vi "estimate_frequency.vi"(4 "FFT Length":i32, 5 "State In":sgl[](array[numeric]), 6 "Prediction Lookahead":sgl, 7 "Central Tip Position (KF)":sgl[](array[numeric])) -> (0 "Prediction":dbl, 1 "State Out":sgl[](array[numeric]), 2 "FFT1":cdb[](array[numeric]), 3 "Xarr":sgl[](array[numeric]))   [LabVIEW 2013]
uses:
  <vilib>/Analysis/2dsp.llb/Real FFT.vi
  <vilib>/Analysis/NI_AALPro.lvlib
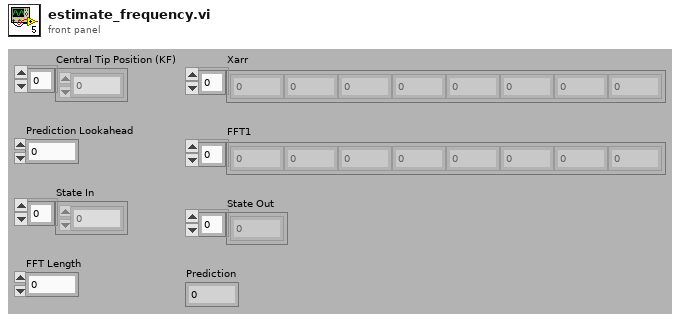
[diagram p1: front panel]
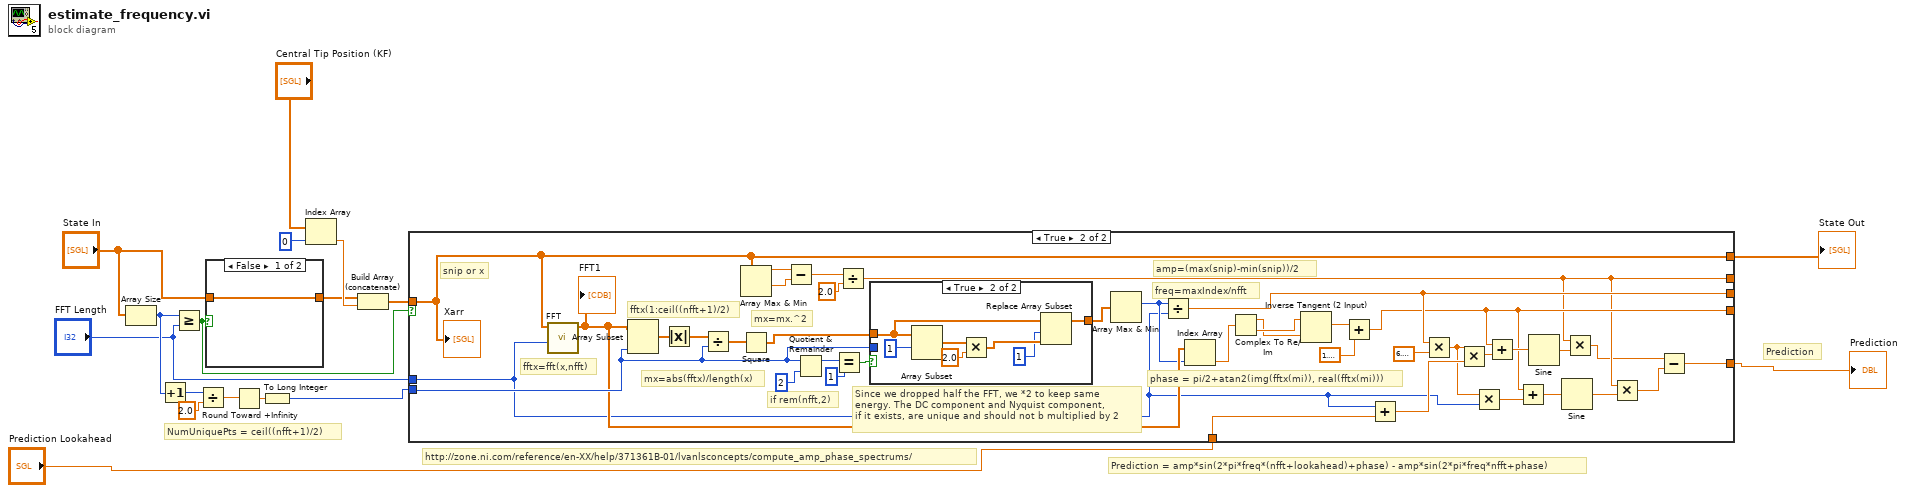
[diagram p0: block diagram]
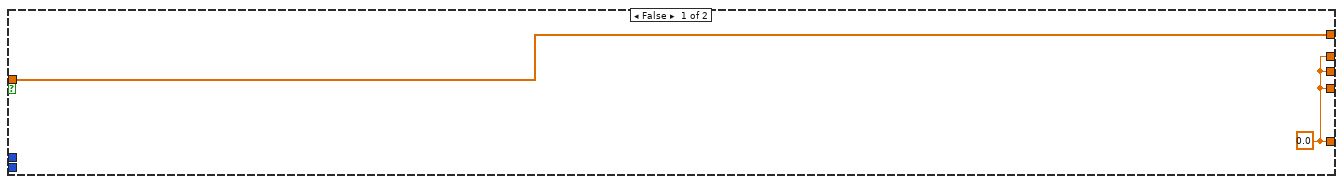
[diagram p2: hidden frame]
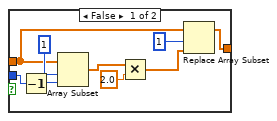
[diagram p3: hidden frame]
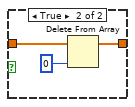
[diagram p4: hidden frame]
diagram:
  # "Prediction = amp*sin(2*pi*freq*(nfft+lookahead)+phase) - amp*sin(2*pi*freq*nfft+phase)"
  # "Prediction"
  # "http://zone.ni.com/reference/en-XX/help/371361B-01/lvanlsconcepts/compute_amp_phase_spectrums/"
  # "NumUniquePts = ceil((nfft+1)/2)"
  n1 = Array Size(array="State In") -> (size(s)=w9:i32)
  n2 = Increment(x=w9) -> (x+1=w10:i32)
  n3 = Greater Or Equal?(x=w9, y="FFT Length") -> (x >= y?=w8:bool)
  n4 = Divide(x=w10, y=sgl 2.0 ("t")) -> (x/y=w12:sgl)
  n5 = case shown="False" w8 {
    tunnel: [w18 w20] -> w2
    tunnel: "State In" -> [w18 w19]
    frame False {
    }
    frame True {
      n6 = Delete From Array(array=w19, index=0 ("t")) -> (array with subset deleted=w20:sgl[])  [unwired: 1 in, 1 out]
    }
  }
  n7 = Round Toward +Infinity(x=w12) -> (ceil(x): smallest int >= x=w13:sgl)
  n8 = To Long Integer(number=w13) -> (32bit integer=w14:i32)
  n9 = Index Array(array="Central Tip Position (KF)", index=0 ("t")) -> (element=w3:sgl)
  n10 = Build Array (concatenate)(w2, w3) -> (w5:sgl[])
  n11 = case shown="True" w8 {
    tunnel: w5 -> [w23 w52]
    tunnel: "FFT Length" -> [_ w33]
    tunnel: [w23 w52] -> w7
    tunnel: w14 -> [_ w54]
    tunnel: [w22 w28] -> _
    tunnel: [w22 w39] -> _
    tunnel: [w22 w31] -> _
    tunnel: [w22 w25] -> w16
    tunnel: "Prediction Lookahead" -> [_ w24]
    frame False {
      w22 = sgl 0.0 ("t")
    }
    frame True {
      # "Since we dropped half the FFT, we *2 to keep same\nenergy. The DC component and Nyquist component,\nif it exists, are unique and should not b multiplied by 2"
      # "phase = pi/2+atan2(img(fftx(mi)), real(fftx(mi)))"
      # "freq=maxIndex/nfft"
      # "snip or x"
      # "amp=(max(snip)-min(snip))/2"
      # "if rem(nfft,2)"
      # "mx=mx.^2"
      # "mx=abs(fftx)/length(x)"
      # "fftx(1:ceil((nfft+1)/2)"
      # "fftx=fft(x,nfft)"
      n12 = call-poly <vilib>:"FFT.vi"("FFT size"=w33, "X"=w52) -> ("FFT {X}"=w47:cdb[])  [unwired: 8 in, 1 out]
      "FFT1" <- w47
      n13 = Array Subset(array=w47, length=w54) -> (w62:cdb[])  [unwired: 1 in]
      n14 = Absolute Value(x=w62) -> (abs(x)=w61:dbl[])
      n15 = Divide(x=w61, y=w54) -> (x/y=w60:dbl[])
      n16 = Array Max & Min(array=w52) -> (max value=w51:sgl, min value=w50:sgl)  [unwired: 2 out]
      n17 = Square(x=w60) -> (x^2=w55:dbl[])
      n18 = Subtract(x=w51, y=w50) -> (x-y=w48:sgl)
      n19 = Quotient & Remainder(x=w54, y=2 ("t")) -> (x-y*floor(x/y)=w58:i32)  [unwired: 1 out]
      n20 = Equal?(x=w58, y=1 ("t")) -> (x = y?=w56:bool)
      n21 = Divide(x=w48, y=sgl 2.0 ("t")) -> (x/y=w28:sgl)
      n22 = case shown="True" w56 {
        tunnel: w55 -> [w65 w75]
        tunnel: w54 -> [w69 _]
        tunnel: [w63 w72] -> w53
        frame False {
          n23 = Decrement(x=w69) -> (x-1=w70:i32)
          n24 = Array Subset(array=w65, index=1 ("t"), length=w70) -> (w68:dbl[])
          n25 = Multiply(x=w68, y=sgl 2.0 ("t")) -> (x*y=w64:dbl[])
          n26 = Replace Array Subset(array=w65, new element=w64, index=1 ("t")) -> (w63:dbl[])
        }
        frame True {
          n27 = Array Subset(array=w75, index=1 ("t")) -> (w77:dbl[])  [unwired: 1 in]
          n28 = Multiply(x=w77, y=sgl 2.0 ("t")) -> (x*y=w74:dbl[])
          n29 = Replace Array Subset(array=w75, new element=w74, index=1 ("t")) -> (w72:dbl[])
        }
      }
      n30 = Array Max & Min(array=w53) -> (max index (indices)=w46:i32)  [unwired: 3 out]
      n31 = Divide(x=w46, y=w33) -> (x/y=w39:dbl)
      n32 = Index Array(array=w47, index=w46) -> (element=w45:cdb)
      n33 = Complex To Re/Im(x + iy=w45) -> (x=w43:dbl, y=w44:dbl)
      n34 = Inverse Tangent (2 Input)(1:w43, 2:w44) -> (0:w42:dbl)
      n35 = Add(x=w42, y=1.5707963267948966) -> (x+y=w31:dbl)
      n36 = Add(x=w33, y=w24) -> (x+y=w38:sgl)
      n37 = Multiply(x=w39, y=6.283185307179586) -> (x*y=w34:dbl)
      n38 = Multiply(x=w34, y=w38) -> (x*y=w37:dbl)
      n39 = Multiply(x=w34, y=w33) -> (x*y=w32:dbl)
      n40 = Add(x=w31, y=w37) -> (x+y=w36:dbl)
      n41 = Add(x=w31, y=w32) -> (x+y=w30:dbl)
      n42 = Sine(x=w36) -> (sin(x)=w35:dbl)
      n43 = Sine(x=w30) -> (sin(x)=w29:dbl)
      n44 = Multiply(x=w28, y=w35) -> (x*y=w27:dbl)
      n45 = Multiply(x=w28, y=w29) -> (x*y=w26:dbl)
      n46 = Subtract(x=w27, y=w26) -> (x-y=w25:dbl)
      "Xarr" <- w52
    }
  }
  "Prediction" <- w16
  "State Out" <- w7
